vi "RFmx_MeasTest_Fetch.vi"(6 "RFmx_Data":refnum<queue>, 7 "Meas_Type":string[](array[string]), 8 "error in (no error)":errorcluster, 11 "Instrument Handle in":refnum<k21>) -> (0 "error out":errorcluster, 3 "Instrument Handle out":refnum<k21>)   [LabVIEW 2014]
uses:
  02_Controls/Message_Data_Ctl.ctl
  <vilib>/RFmx/RFInstr/mx/RFmxInstr.llb/RFmxInstr Build Signal String.vi
  <vilib>/RFmx/SpecAn/mx/RFmxSpecAn.llb/RFmxSpecAn Spectrum Fetch Measurement.vi
  <vilib>/RFmx/SpecAn/mx/RFmxSpecAn.llb/RFmxSpecAn Spectrum Fetch Spectrum.vi
  <vilib>/RFmx/SpecAn/mx/RFmxSpecAn.llb/RFmxSpecAn ACP Fetch Total Carrier Power.vi
  <vilib>/RFmx/SpecAn/mx/RFmxSpecAn.llb/RFmxSpecAn ACP Fetch Offset Measurement (Array).vi
  <vilib>/RFmx/SpecAn/mx/RFmxSpecAn.llb/RFmxSpecAn ACP Fetch Spectrum.vi
  <vilib>/RFmx/SpecAn/mx/RFmxSpecAn.llb/RFmxSpecAn CHP Fetch Total Carrier Power.vi
  <vilib>/RFmx/SpecAn/mx/RFmxSpecAn.llb/RFmxSpecAn CHP Fetch Spectrum.vi
  <vilib>/RFmx/SpecAn/mx/RFmxSpecAn.llb/RFmxSpecAn OBW Fetch Measurement.vi
  <vilib>/RFmx/SpecAn/mx/RFmxSpecAn.llb/RFmxSpecAn OBW Fetch Spectrum Trace.vi
  <vilib>/RFmx/SpecAn/mx/RFmxSpecAn.llb/RFmxSpecAn TXP Fetch Measurement.vi
  <vilib>/RFmx/SpecAn/mx/RFmxSpecAn.llb/RFmxSpecAn TXP Fetch Power Trace.vi
  <vilib>/RFmx/SpecAn/mx/RFmxSpecAn.llb/RFmxSpecAn CCDF Fetch Power.vi
  <vilib>/RFmx/SpecAn/mx/RFmxSpecAn.llb/RFmxSpecAn CCDF Fetch Probabilities Trace.vi
  <vilib>/RFmx/SpecAn/mx/RFmxSpecAn.llb/RFmxSpecAn CCDF Fetch Gaussian Probabilities Trace.vi
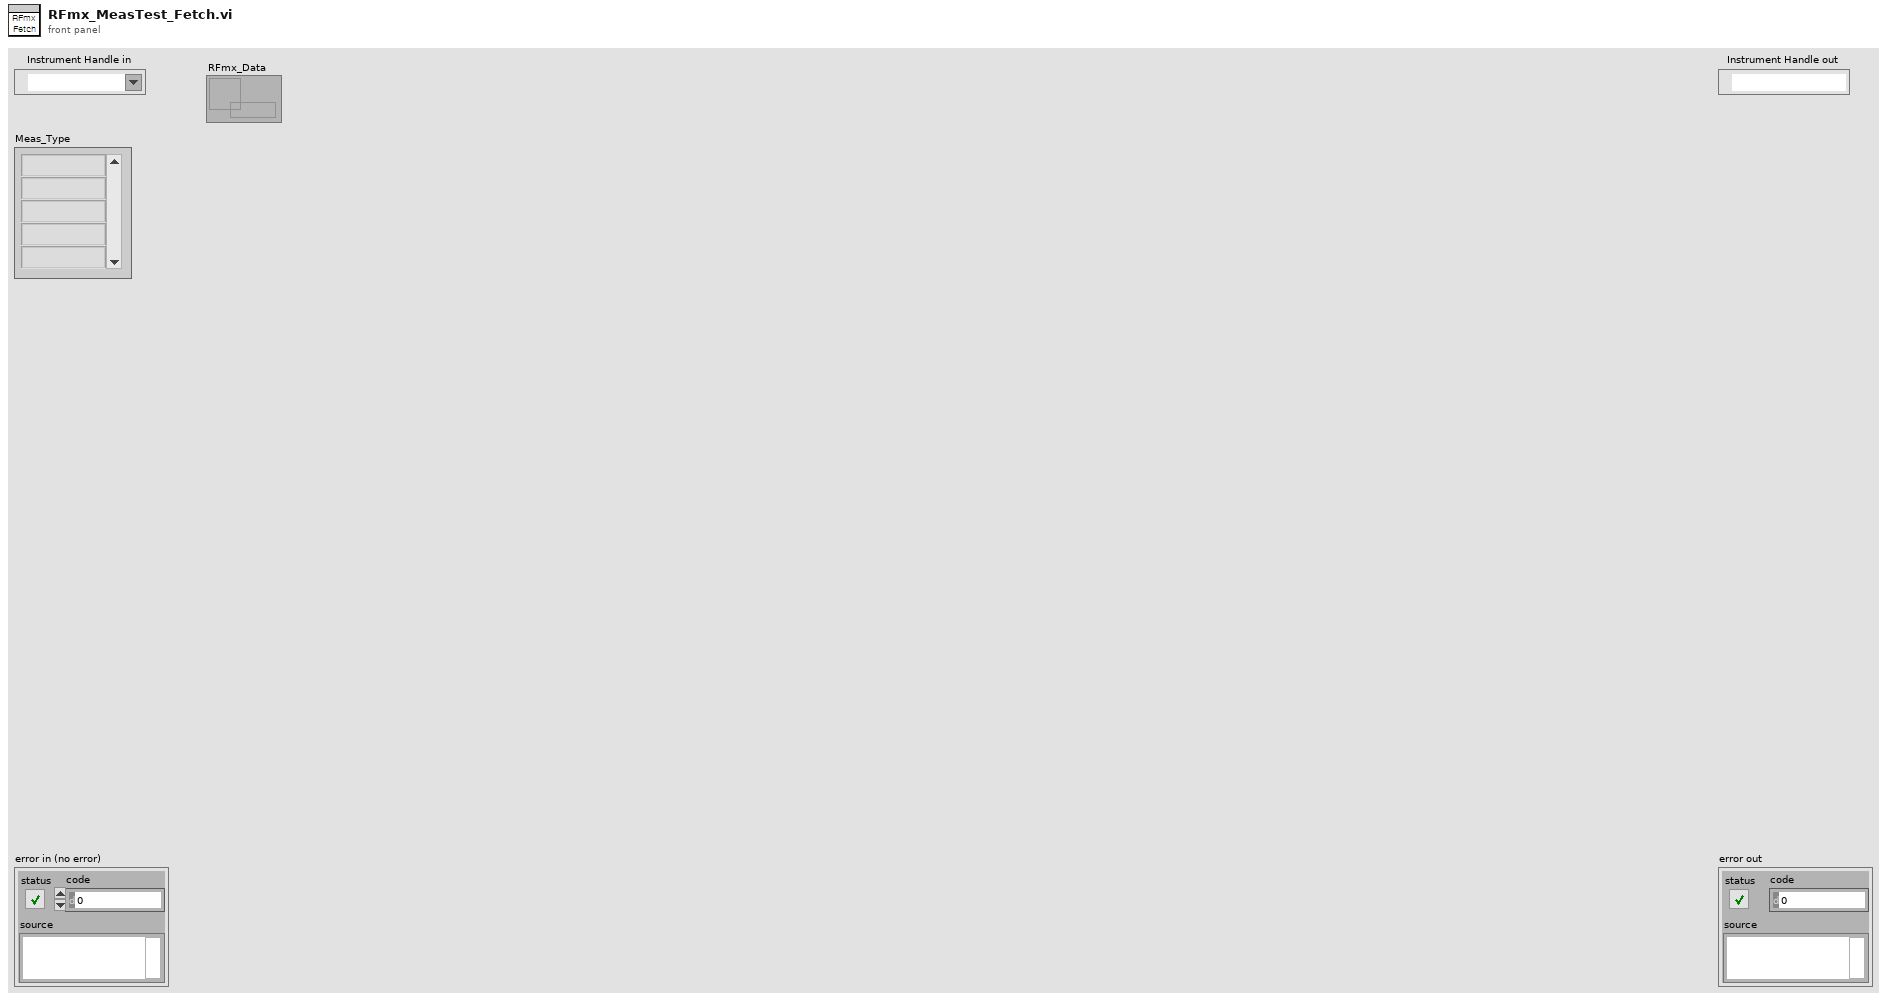
[diagram p1: front panel]
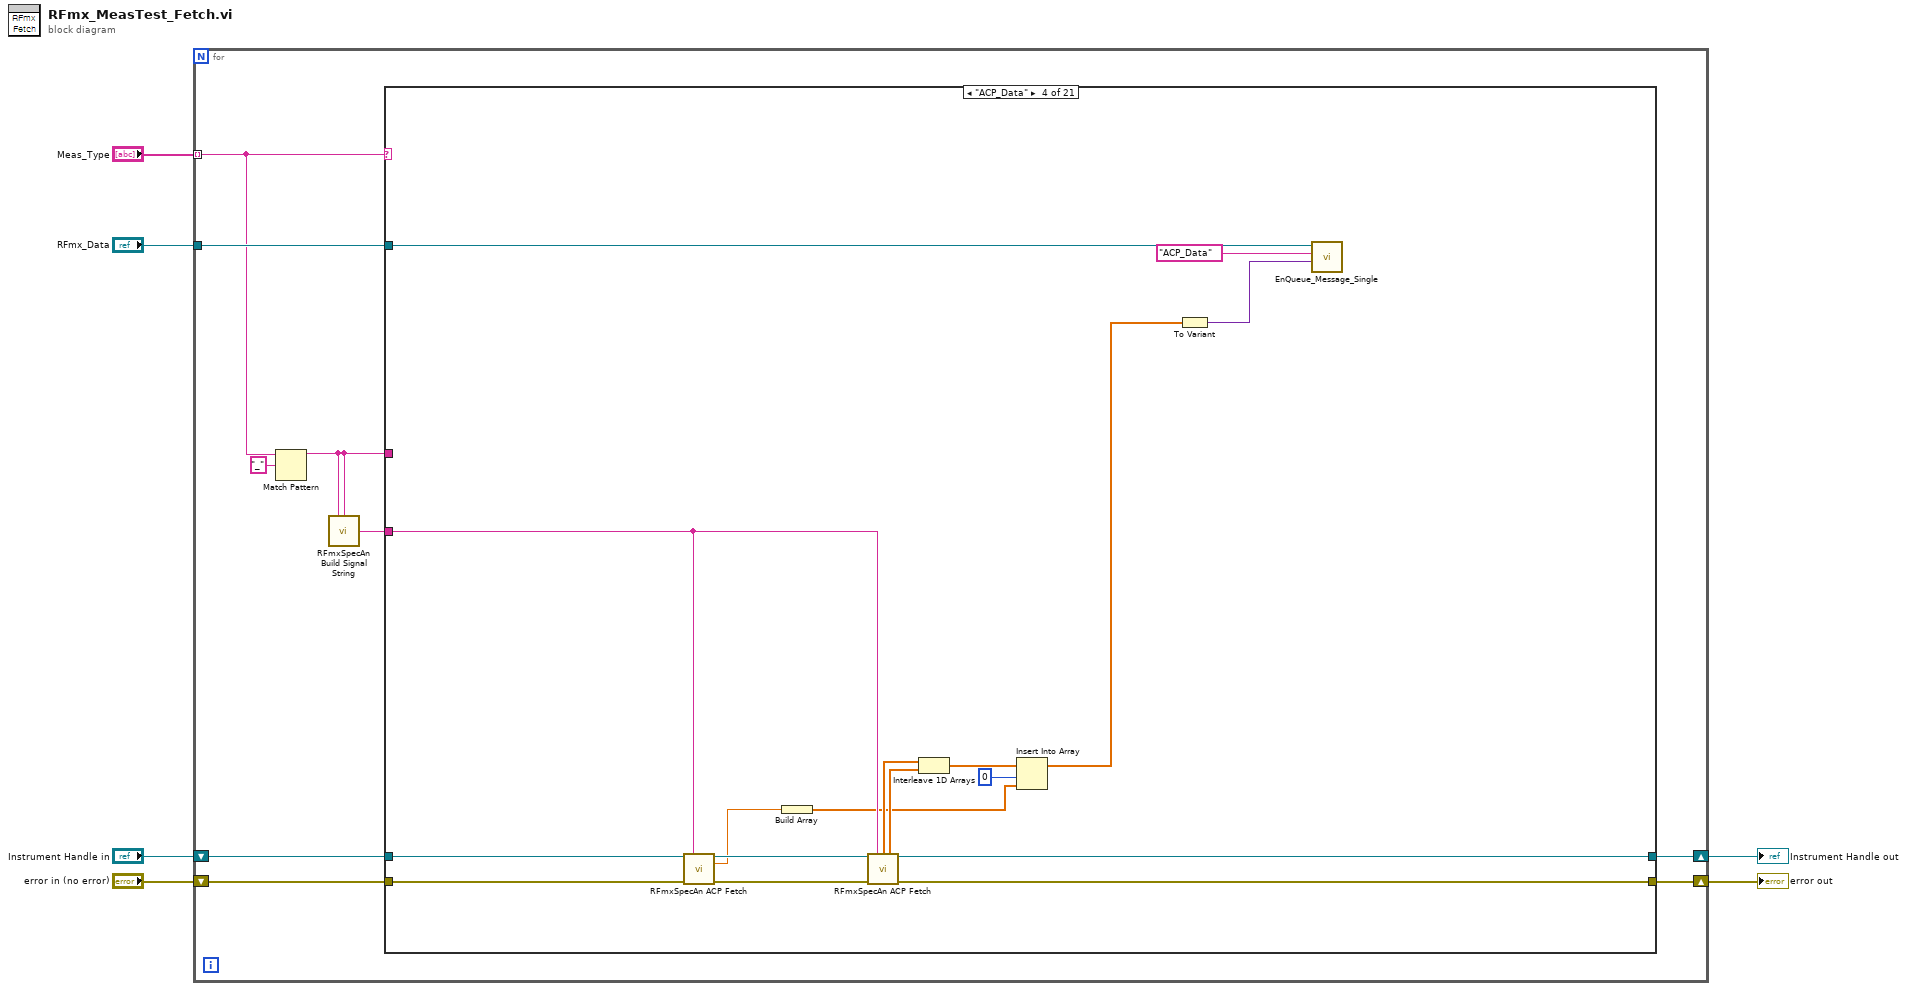
[diagram p0: block diagram]
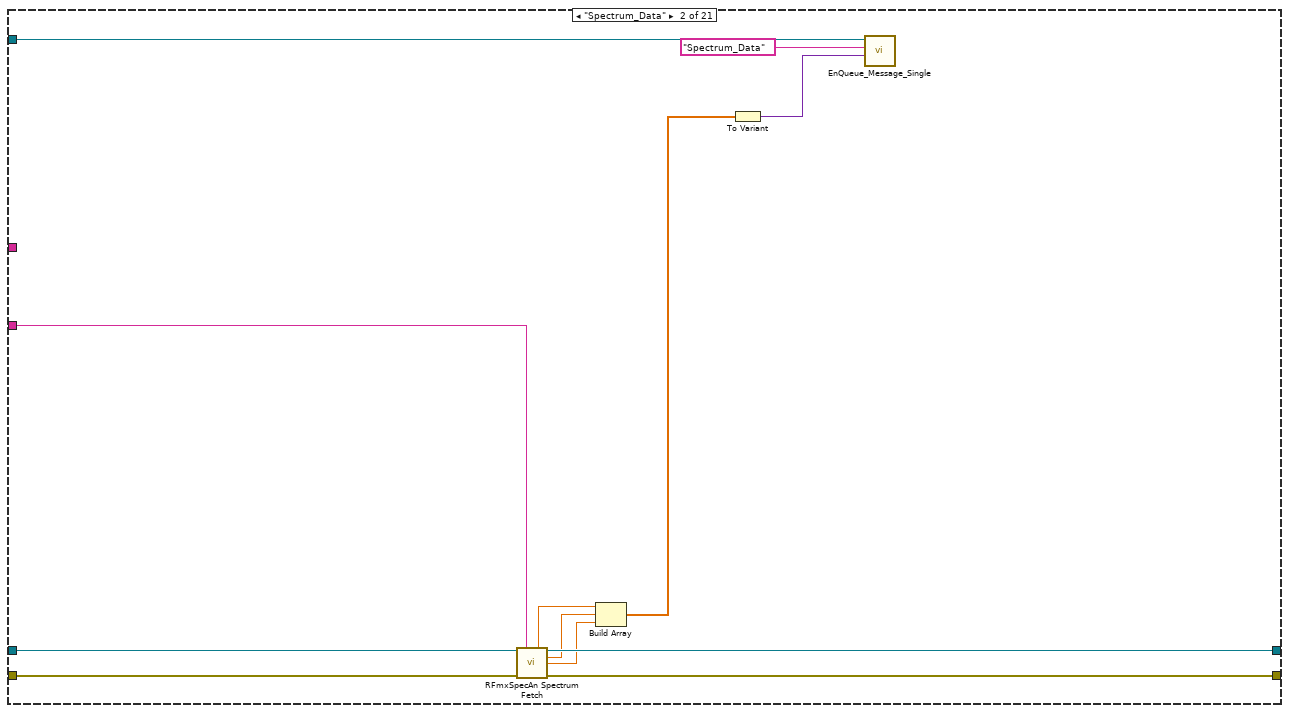
[diagram p3: hidden frame]
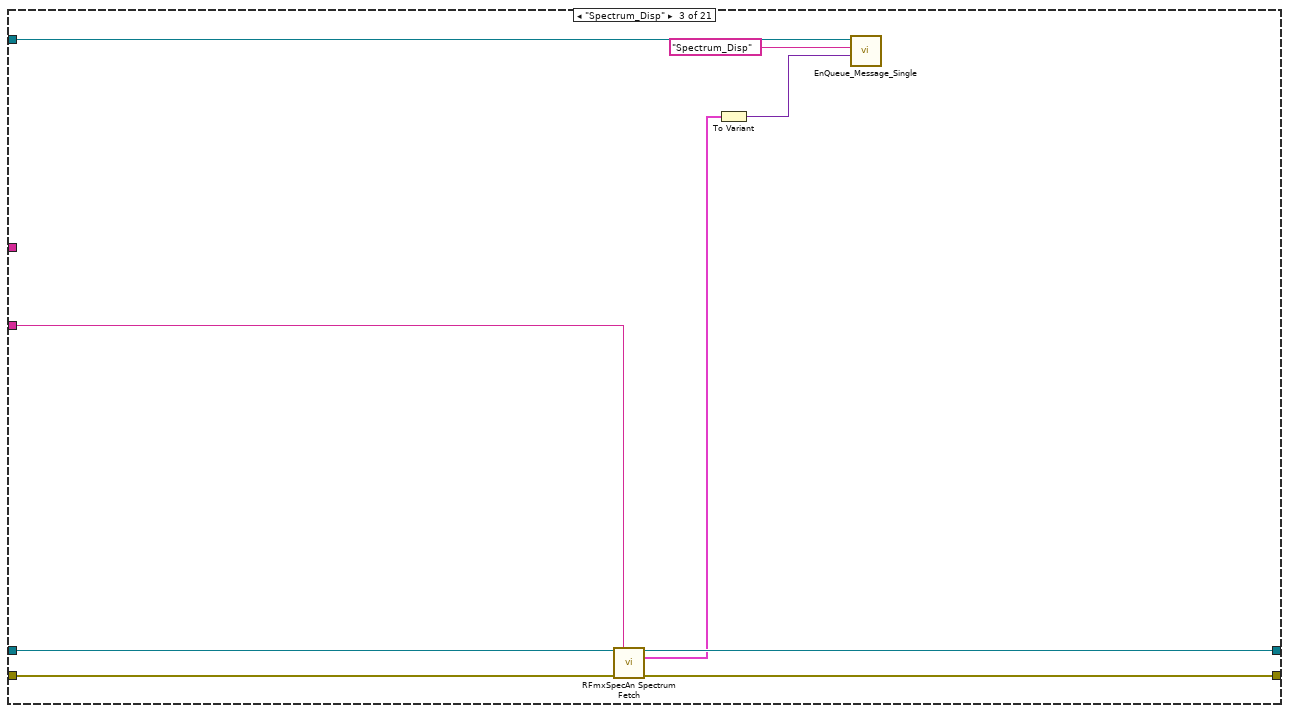
[diagram p4: hidden frame]
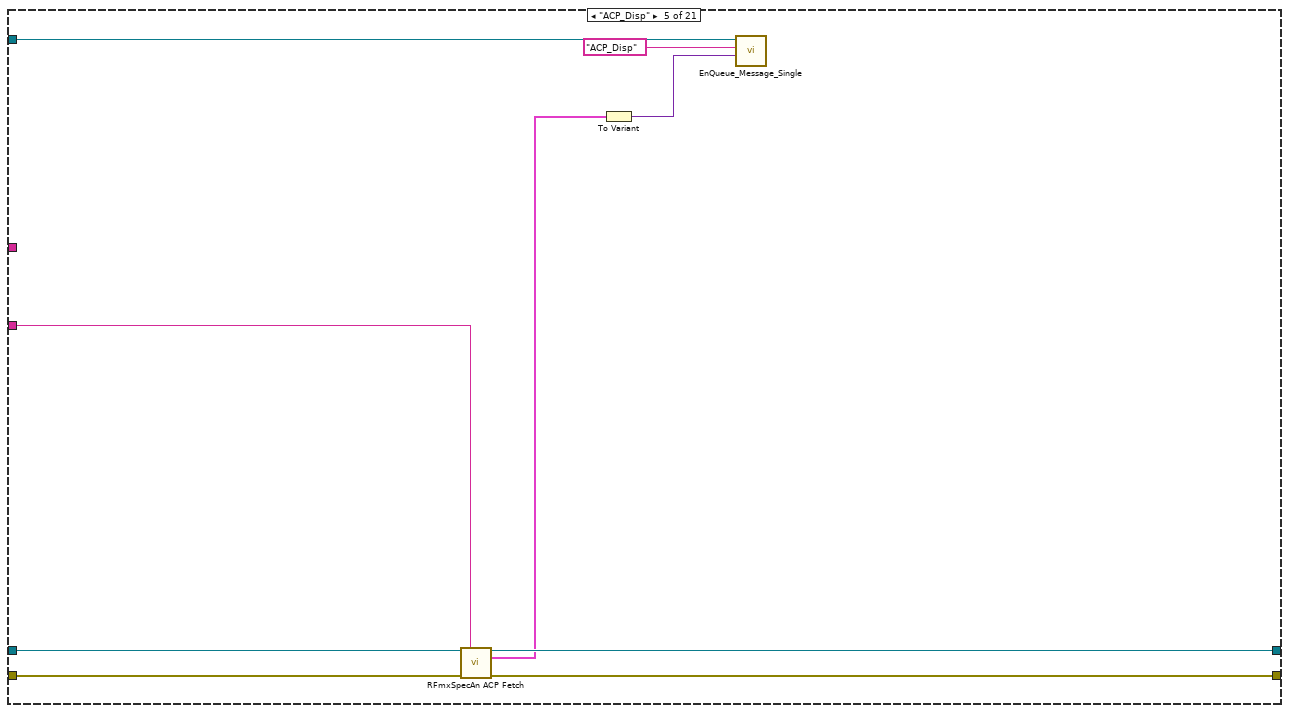
[diagram p5: hidden frame]
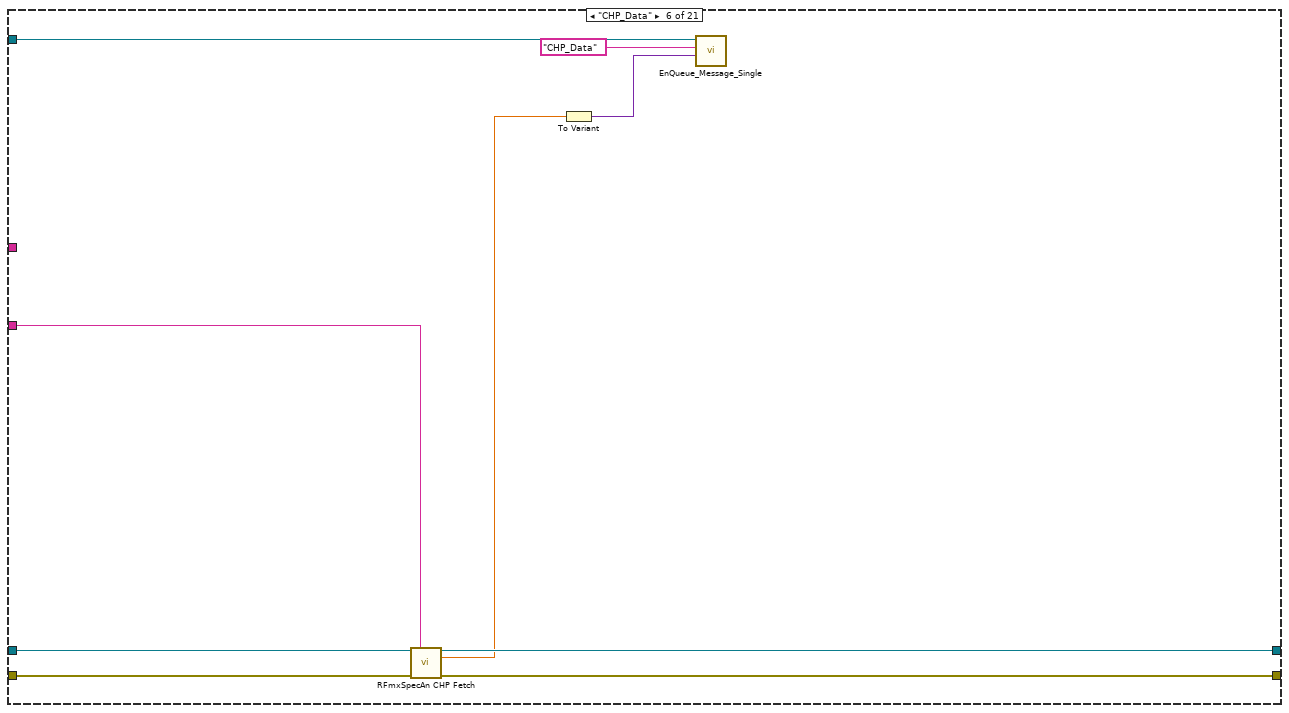
[diagram p6: hidden frame]
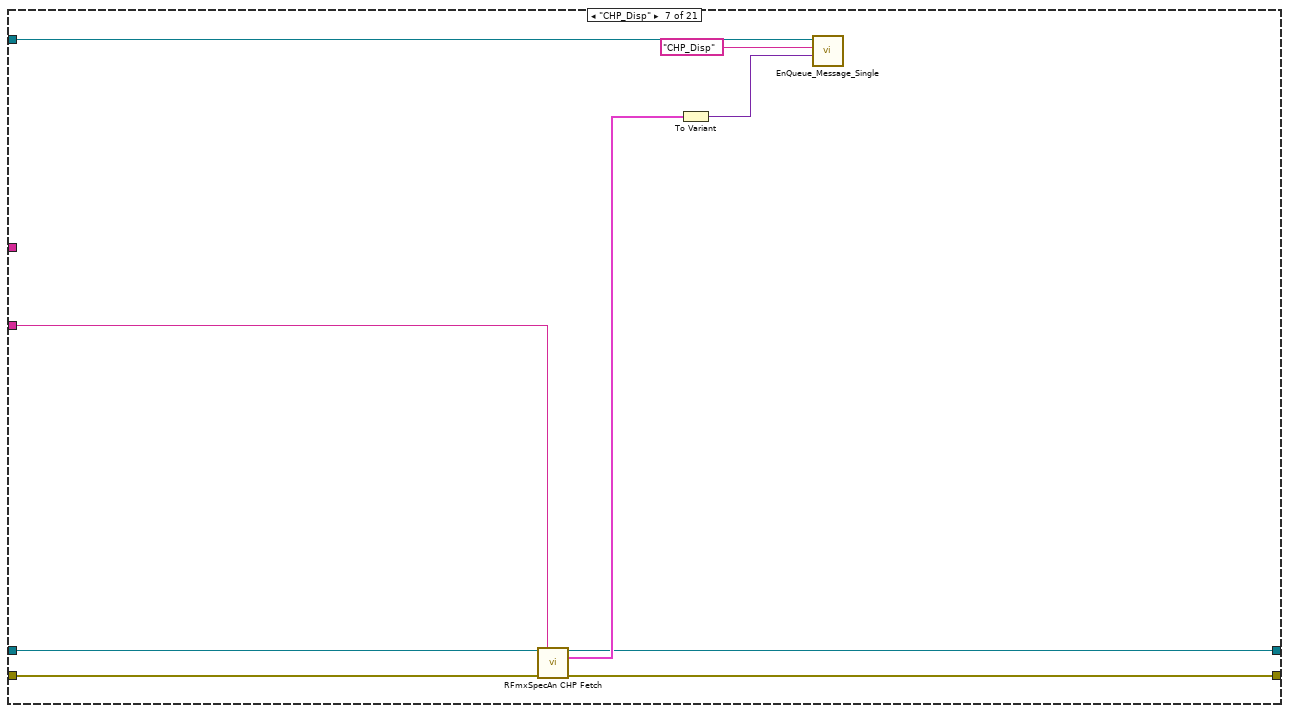
[diagram p7: hidden frame]
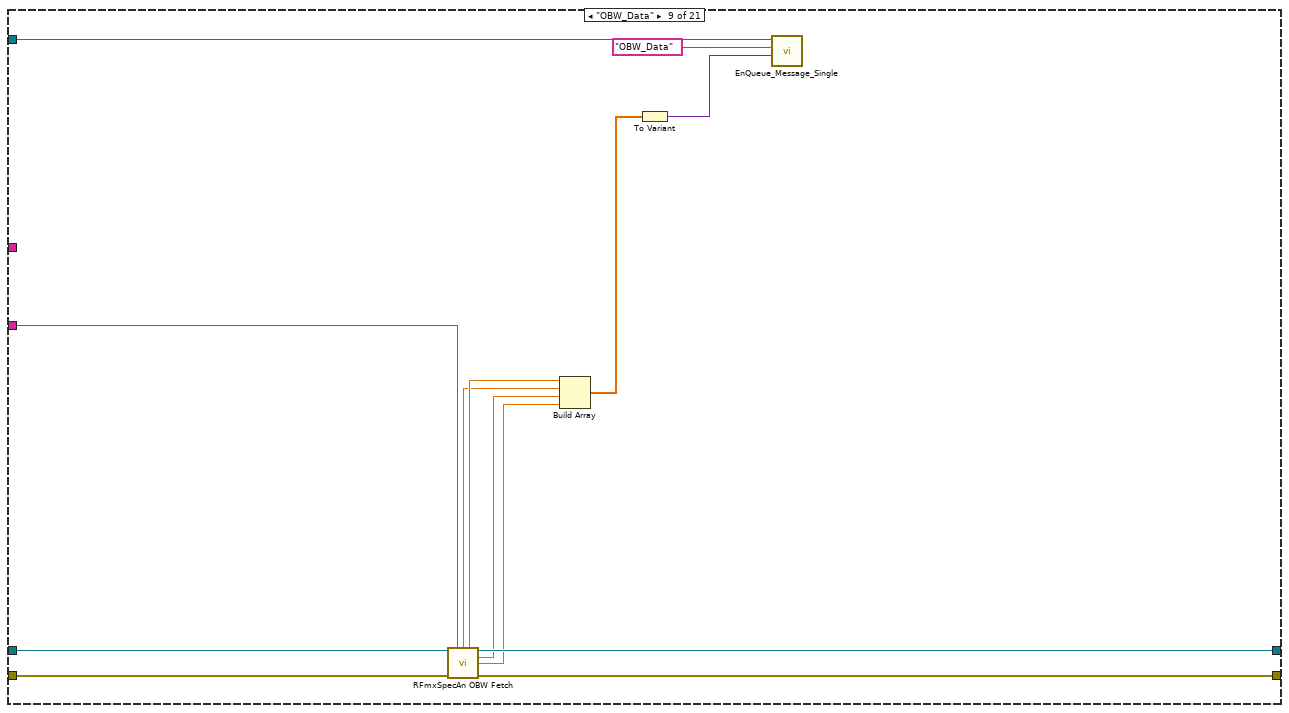
[diagram p9: hidden frame]
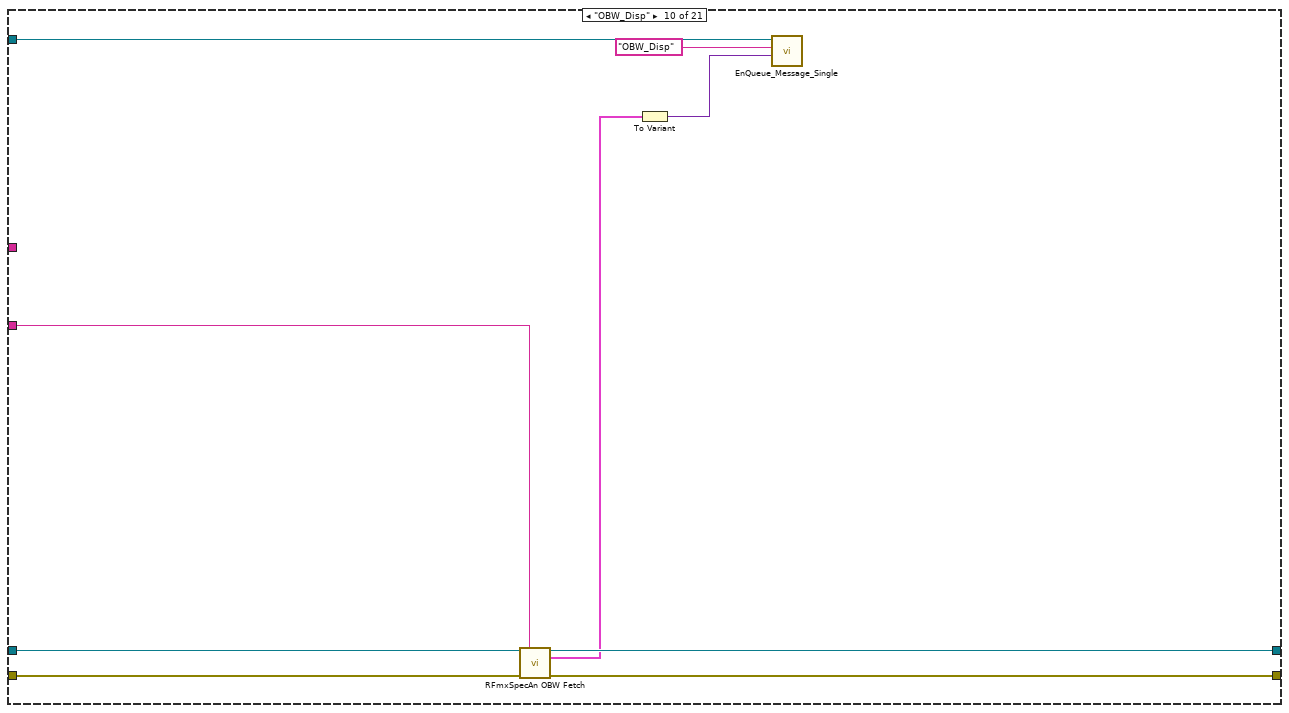
[diagram p10: hidden frame]
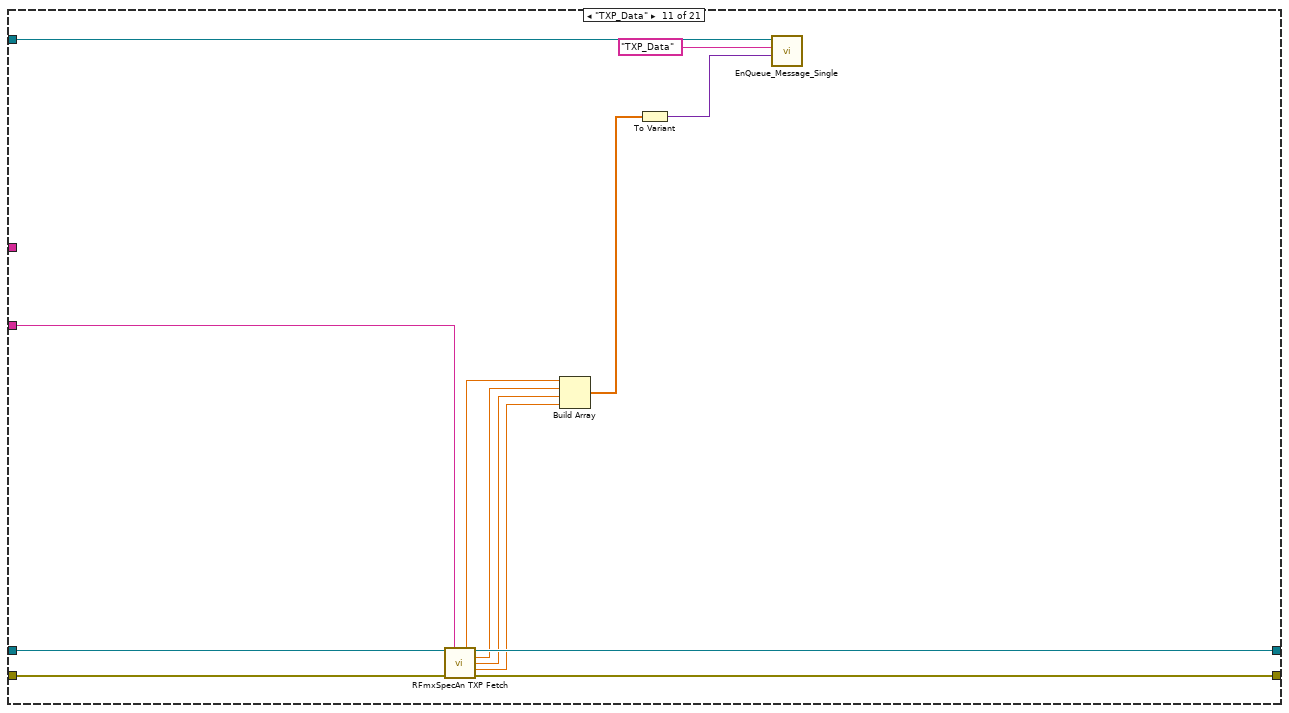
[diagram p11: hidden frame]
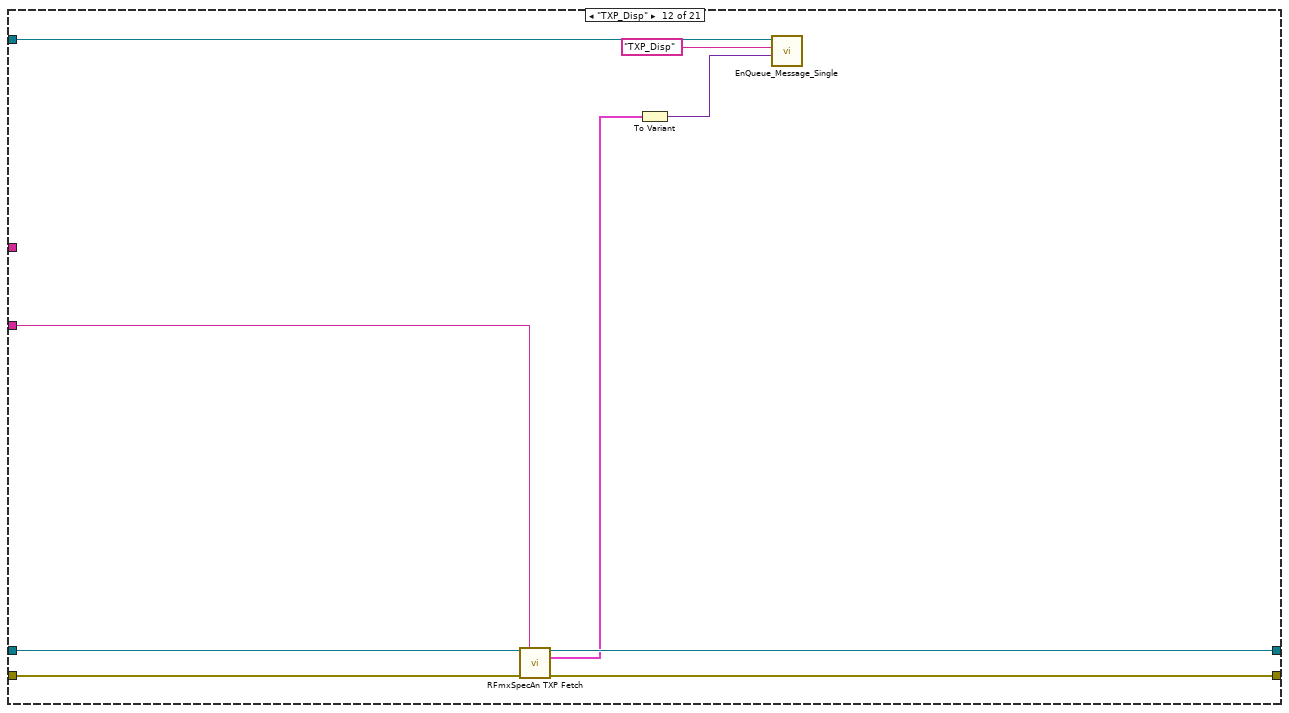
[diagram p12: hidden frame]
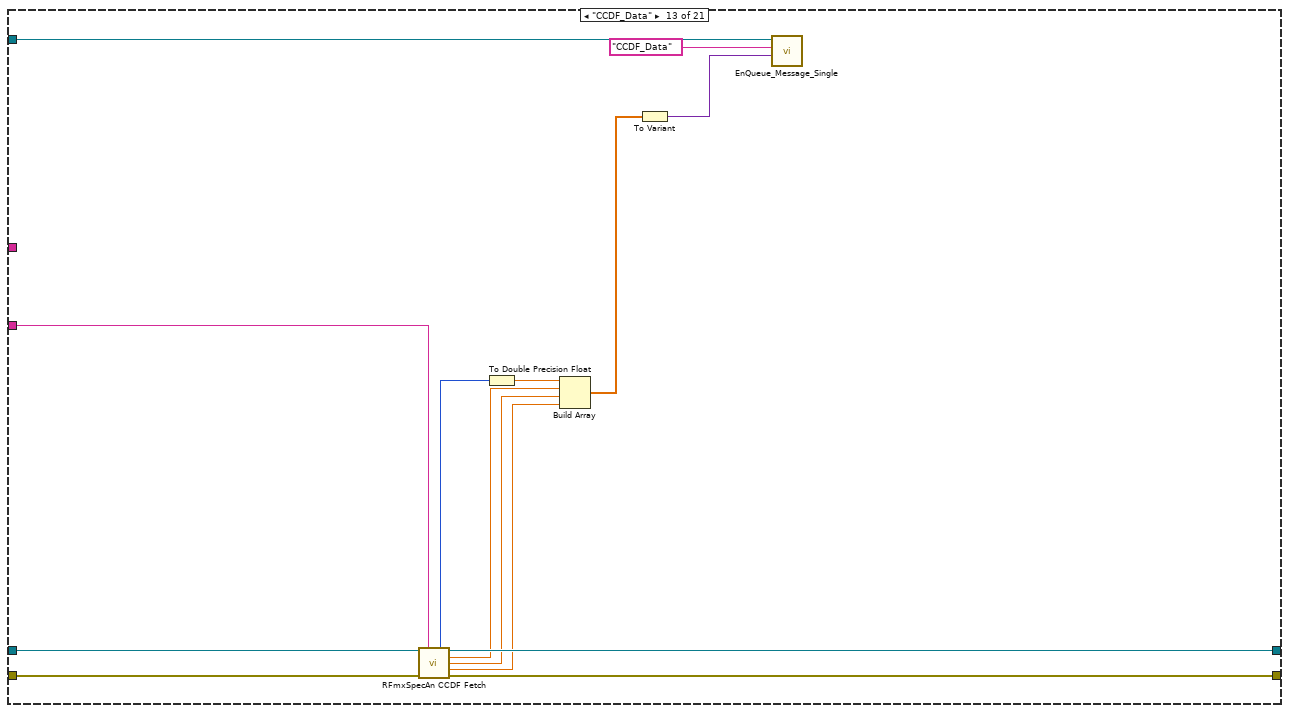
[diagram p13: hidden frame]
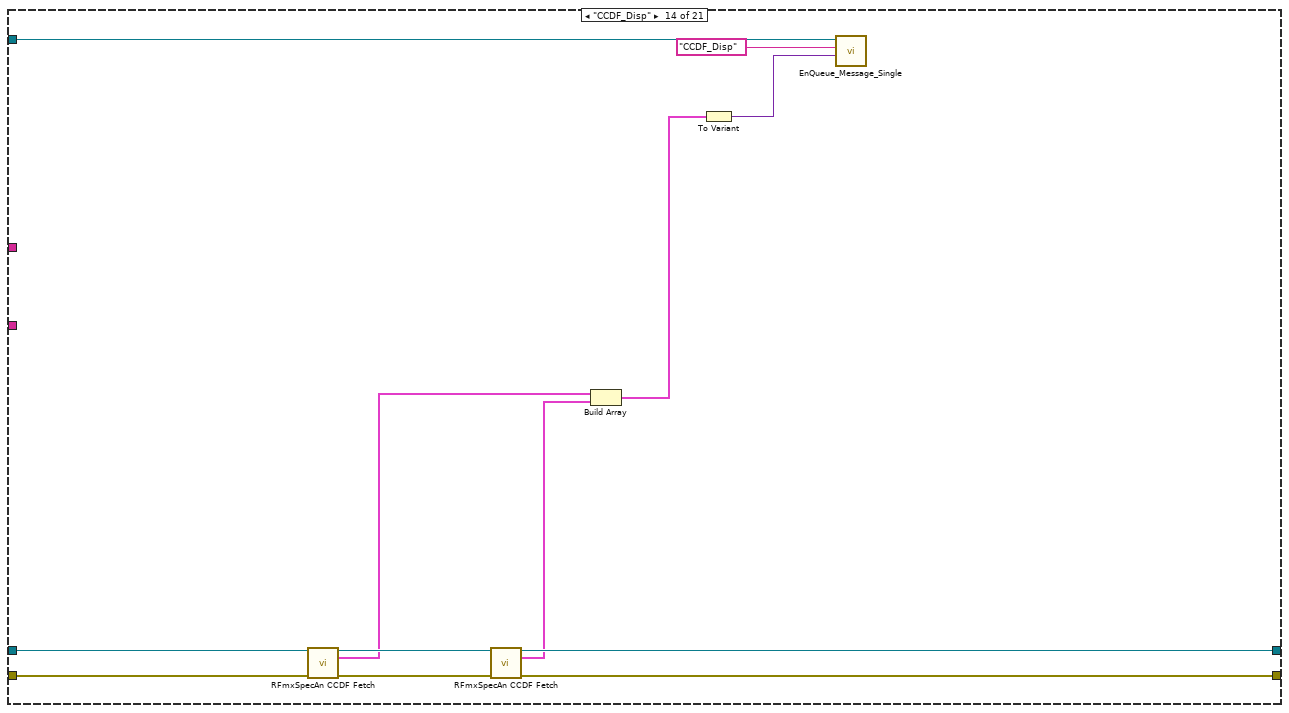
[diagram p14: hidden frame]
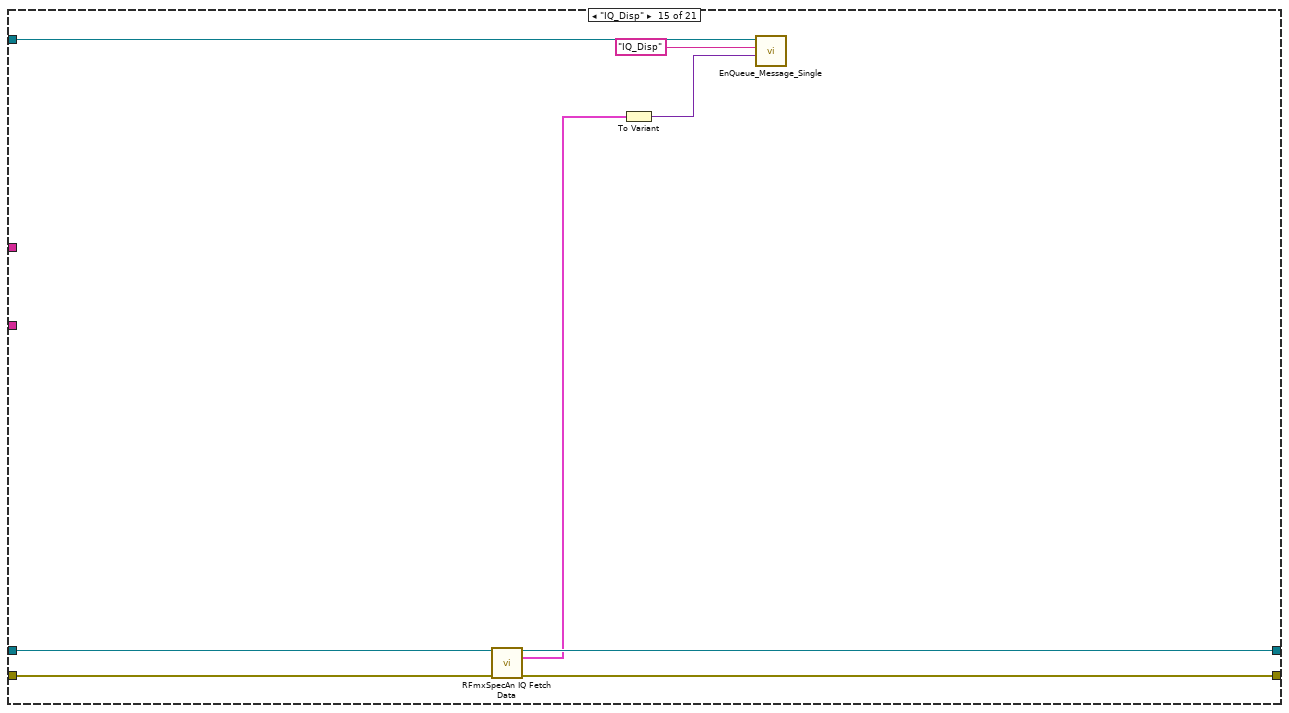
[diagram p15: hidden frame]
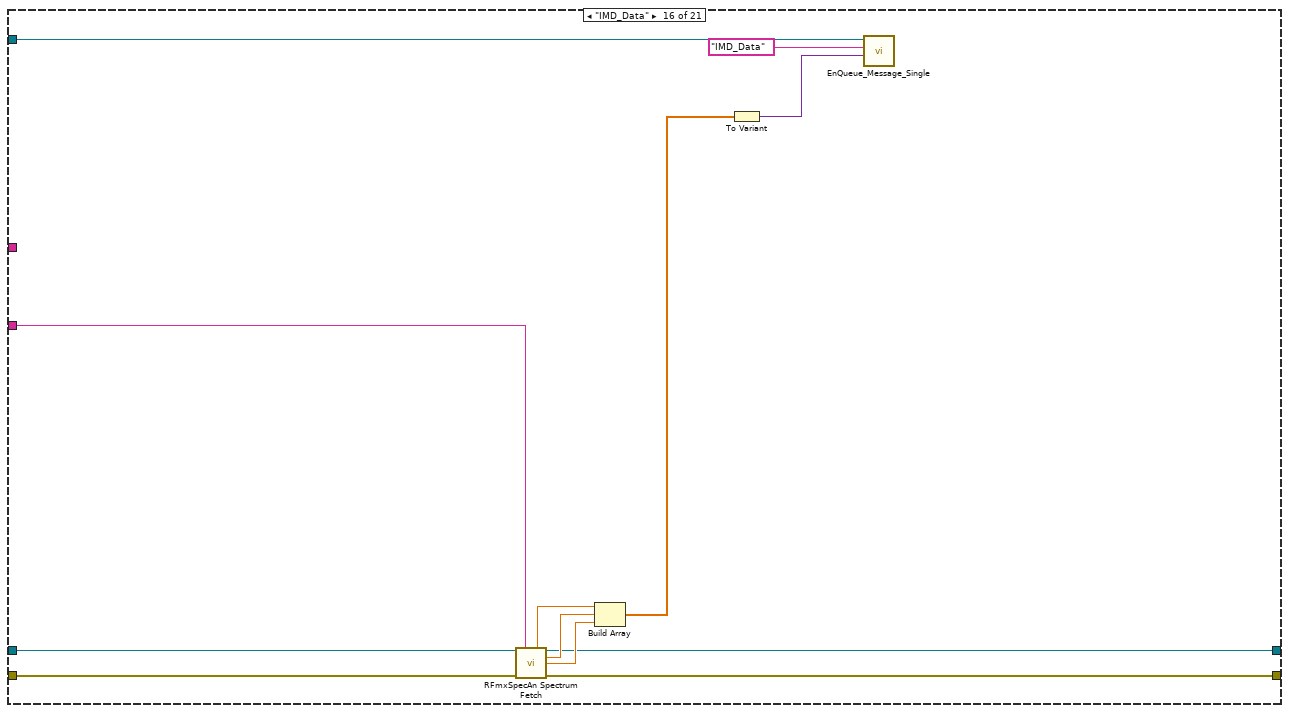
[diagram p16: hidden frame]
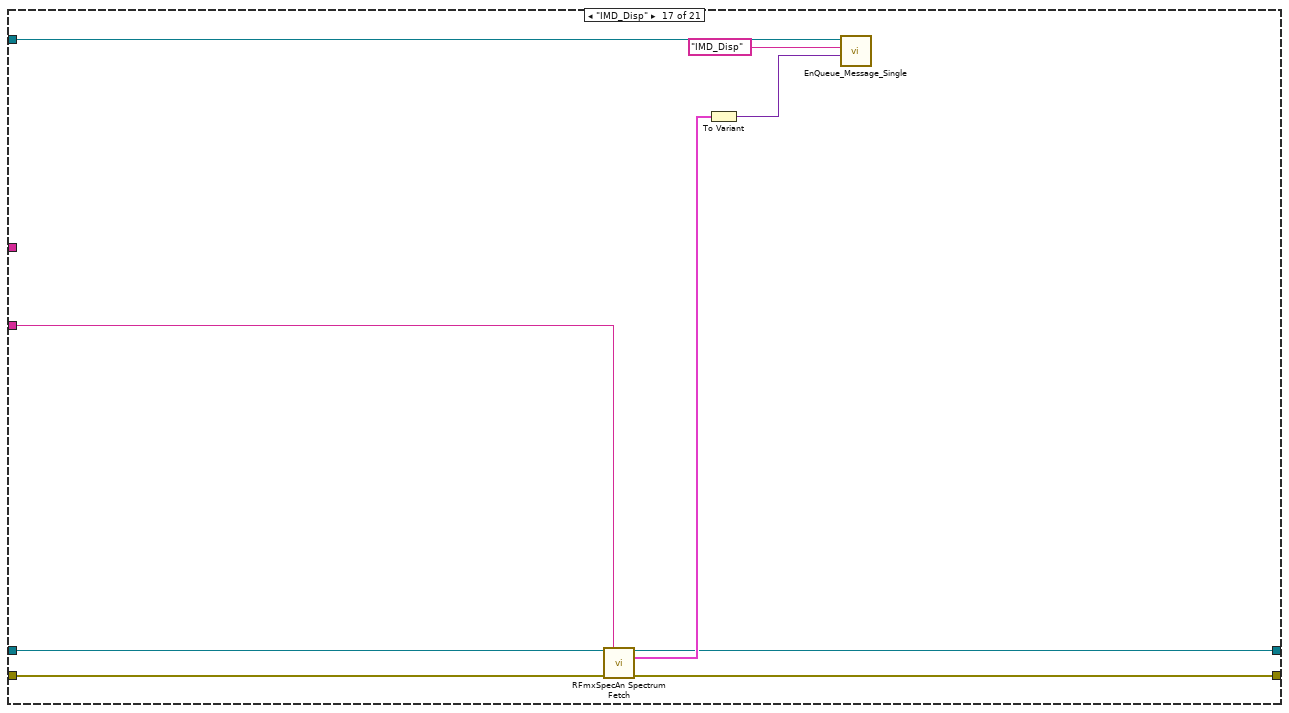
[diagram p17: hidden frame]
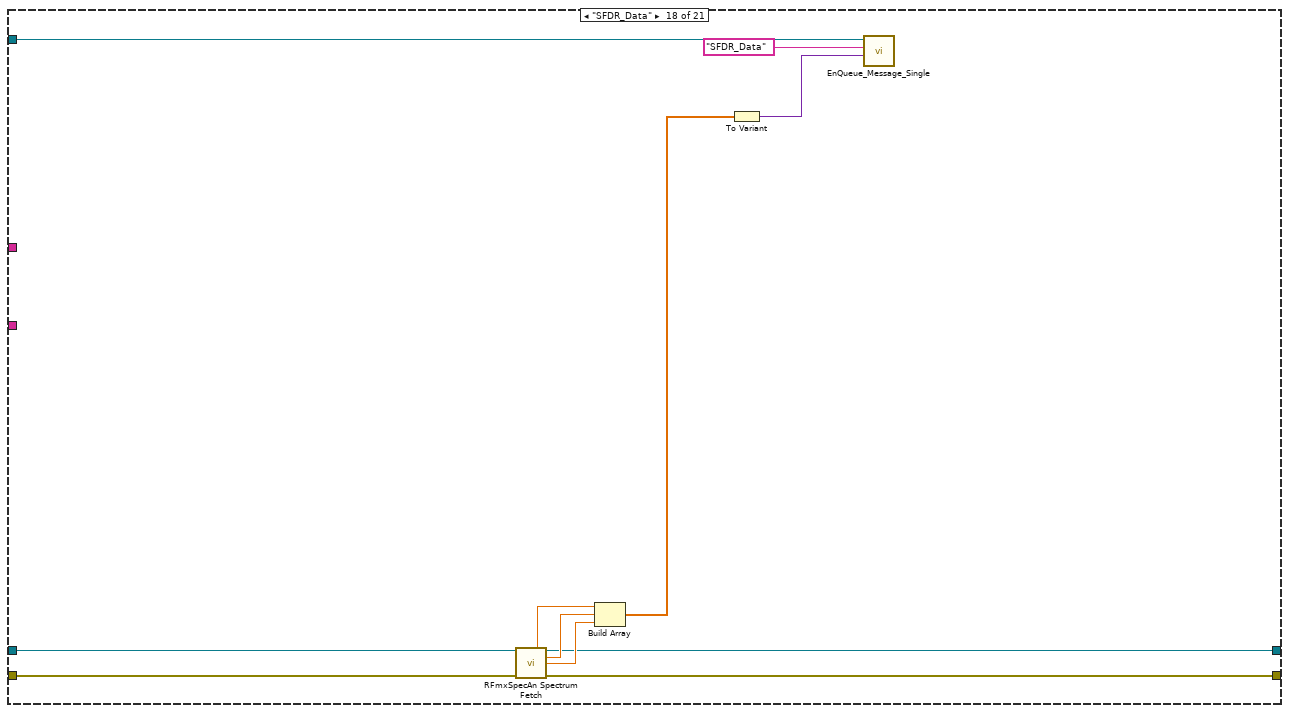
[diagram p18: hidden frame]
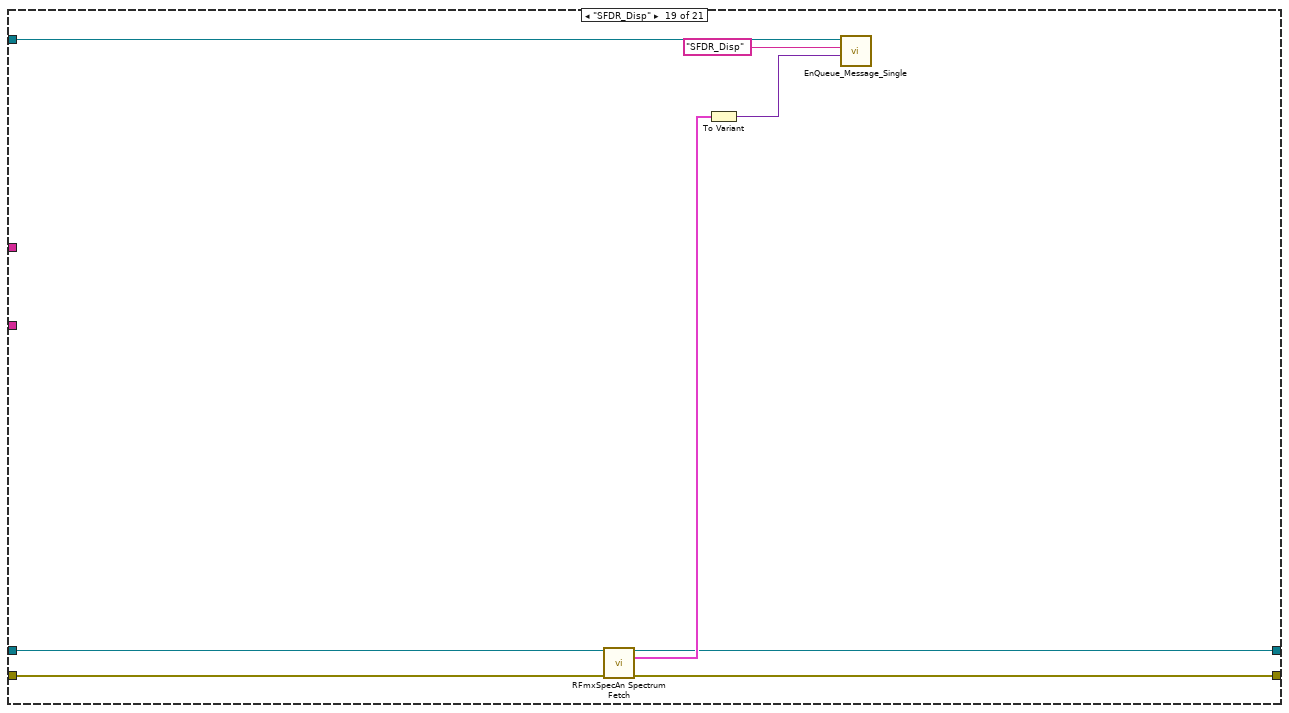
[diagram p19: hidden frame]
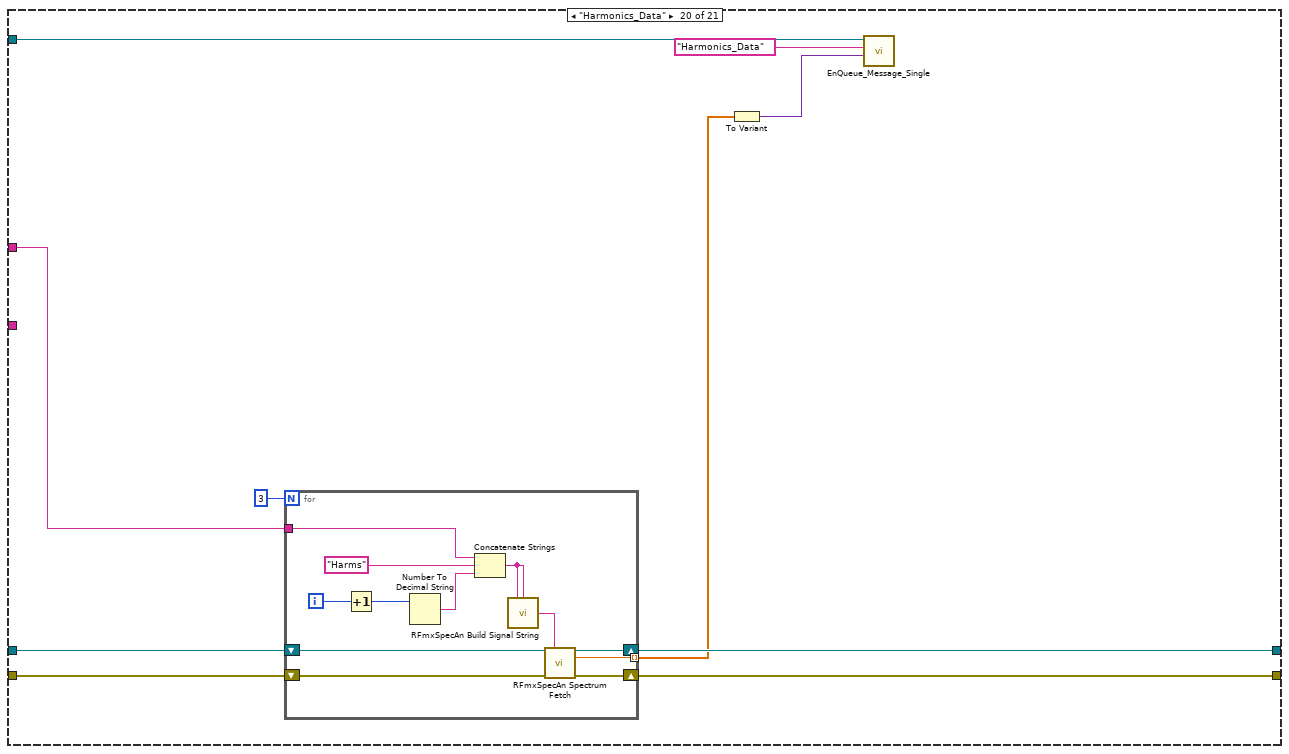
[diagram p20: hidden frame]
diagram:
  n1 = for {
    tunnel: "RFmx_Data" -> [w11]
    shift-right: [w12] -> w3
    shift-left: "Instrument Handle in" -> [w15]
    shift-right: [w13] -> w4
    shift-left: "error in (no error)" -> [w14]
    tunnel: "Meas_Type" -> [w8] mode=indexing
    n2 = Match Pattern(string=w8, regular expression="_") -> (before substring=w7:string)  [unwired: 1 in, 3 out]
    n3 = call <vilib>:"RFmxSpecAn Build Signal String.vi"("Signal Name"=w7, "Result Name"=w7) -> ("Selector String"=w10:string)  [unwired: 13 in]
    n4 = case shown="\"ACP_Data\"" w8 {
      tunnel: w15 -> [w17 w29 w38 w54 w58 w68 w79 w84 w97 w106 w115 w128 w138 w149 w162 w168 w180 w188 w199 w207 w230]
      tunnel: w14 -> [w16 w28 w37 w53 w57 w67 w78 w83 w96 w105 w114 w127 w137 w148 w161 w167 w179 w187 w198 w206 w229]
      tunnel: [w17 w27 w36 w50 w64 w70 w76 w84 w95 w104 w112 w126 w135 w151 w160 w166 w177 w186 w196 w205 w228] -> w12
      tunnel: [w16 w26 w35 w49 w63 w69 w77 w83 w94 w103 w113 w125 w136 w150 w159 w165 w176 w185 w195 w204 w227] -> w13
      tunnel: w11 -> [_ w23 w31 w55 w61 w73 w75 _ w91 w100 w117 w122 w140 w152 w156 w164 w178 w184 w197 w210 w232]
      tunnel: w10 -> [_ w18 w30 w41 w56 w65 w74 _ w85 w98 w107 w120 w129 _ _ w163 w175 _ _ _ _]
      tunnel: w7 -> [_ _ _ _ _ _ _ _ _ _ _ _ _ _ _ _ _ _ _ w208 w226]
      frame "Nothing", Default {
      }
      frame "Spectrum_Data" {
        n5 = call-poly <vilib>:"RFmxSpecAn Spectrum Fetch.vi"("Instrument Handle In"=w29, "Selector String"=w18, "error in (no error)"=w28) -> ("Frequency Resolution (Hz)"=w22:dbl, "Instrument Handle Out"=w27:refnum<k21>, "Peak Amplitude"=w21:dbl, "Peak Frequency (Hz)"=w20:dbl, "error out"=w26:errorcluster)  [unwired: 8 in]
        n6 = Build Array(w22, w21, w20) -> (w19:dbl[])
        n7 = To Variant(anything=w19) -> (Variant=w25:variant)
        n8 = call "EnQueue_Message_Single.vi"("Message Data"=w25, "Message"="Spectrum_Data", "Message_Queue"=w23) -> ()  [unwired: 7 in, 2 out]
      }
      frame "Spectrum_Disp" {
        n9 = call-poly <vilib>:"RFmxSpecAn Spectrum Fetch.vi"("Instrument Handle In"=w38, "Selector String"=w30, "error in (no error)"=w37) -> ("Instrument Handle Out"=w36:refnum<k21>, "Spectrum"=w32:cluster{"x0":dbl, "dx":dbl, "y":sgl[]}, "error out"=w35:errorcluster)  [unwired: 10 in]
        n10 = To Variant(anything=w32) -> (Variant=w34:variant)
        n11 = call "EnQueue_Message_Single.vi"("Message Data"=w34, "Message"="Spectrum_Disp", "Message_Queue"=w31) -> ()  [unwired: 7 in, 2 out]
      }
      frame "ACP_Data" {
        n12 = call-poly <vilib>:"RFmxSpecAn ACP Fetch.vi"("Instrument Handle In"=w54, "Selector String"=w41, "error in (no error)"=w53) -> ("Instrument Handle Out"=w52:refnum<k21>, "Total Carrier Power (dBm or dBm/Hz)"=w44:dbl, "error out"=w51:errorcluster)  [unwired: 10 in]
        n13 = Build Array(w44) -> (w39:dbl[])
        n14 = call-poly <vilib>:"RFmxSpecAn ACP Fetch.vi"("Instrument Handle In"=w52, "Selector String"=w41, "error in (no error)"=w51) -> ("Lower Absolute Power (dBm or dBm/Hz)"=w46:dbl[], "Upper Absolute Power (dBm or dBm/Hz)"=w45:dbl[], "Instrument Handle Out"=w50:refnum<k21>, "error out"=w49:errorcluster)  [unwired: 7 in, 2 out]
        n15 = Interleave 1D Arrays(w46, w45) -> (w40:dbl[])
        n16 = Insert Into Array(array=w40, index=0, new element=w39) -> (w42:dbl[])
        n17 = To Variant(anything=w42) -> (Variant=w48:variant)
        n18 = call "EnQueue_Message_Single.vi"("Message Data"=w48, "Message"="ACP_Data", "Message_Queue"=w55) -> ()  [unwired: 7 in, 2 out]
      }
      frame "ACP_Disp" {
        n19 = call-poly <vilib>:"RFmxSpecAn ACP Fetch.vi"("Instrument Handle In"=w58, "Selector String"=w56, "error in (no error)"=w57) -> ("Instrument Handle Out"=w64:refnum<k21>, "Spectrum (dBm or dBm/Hz)"=w62:cluster{"x0":dbl, "dx":dbl, "y":sgl[]}, "error out"=w63:errorcluster)  [unwired: 10 in]
        n20 = To Variant(anything=w62) -> (Variant=w60:variant)
        n21 = call "EnQueue_Message_Single.vi"("Message Data"=w60, "Message"="ACP_Disp", "Message_Queue"=w61) -> ()  [unwired: 7 in, 2 out]
      }
      frame "CHP_Data" {
        n22 = call-poly <vilib>:"RFmxSpecAn CHP Fetch.vi"("Instrument Handle In"=w68, "Selector String"=w65, "error in (no error)"=w67) -> ("Instrument Handle Out"=w70:refnum<k21>, "Total Carrier Power (dBm)"=w66:dbl, "error out"=w69:errorcluster)  [unwired: 10 in]
        n23 = To Variant(anything=w66) -> (Variant=w72:variant)
        n24 = call "EnQueue_Message_Single.vi"("Message Data"=w72, "Message"="CHP_Data", "Message_Queue"=w73) -> ()  [unwired: 7 in, 2 out]
      }
      frame "CHP_Disp" {
        n25 = call-poly <vilib>:"RFmxSpecAn CHP Fetch.vi"("Instrument Handle In"=w79, "Selector String"=w74, "error in (no error)"=w78) -> ("Instrument Handle Out"=w76:refnum<k21>, "Spectrum (dBm)"=w82:cluster{"x0":dbl, "dx":dbl, "y":sgl[]}, "error out"=w77:errorcluster)  [unwired: 10 in]
        n26 = To Variant(anything=w82) -> (Variant=w81:variant)
        n27 = call "EnQueue_Message_Single.vi"("Message Data"=w81, "Message"="CHP_Disp", "Message_Queue"=w75) -> ()  [unwired: 7 in, 2 out]
      }
      frame "FCnt" {
      }
      frame "OBW_Data" {
        n28 = call-poly <vilib>:"RFmxSpecAn OBW Fetch.vi"("Instrument Handle In"=w97, "Selector String"=w85, "error in (no error)"=w96) -> ("Stop Frequency (Hz)"=w89:dbl, "Start Frequency (Hz)"=w90:dbl, "Instrument Handle Out"=w95:refnum<k21>, "Occupied Bandwidth (Hz)"=w88:dbl, "Average Power (dBm or dBm/Hz)"=w87:dbl, "error out"=w94:errorcluster)  [unwired: 6 in, 1 out]
        n29 = Build Array(w90, w89, w88, w87) -> (w86:dbl[])
        n30 = To Variant(anything=w86) -> (Variant=w93:variant)
        n31 = call "EnQueue_Message_Single.vi"("Message Data"=w93, "Message"="OBW_Data", "Message_Queue"=w91) -> ()  [unwired: 7 in, 2 out]
      }
      frame "OBW_Disp" {
        n32 = call-poly <vilib>:"RFmxSpecAn OBW Fetch.vi"("Instrument Handle In"=w106, "Selector String"=w98, "error in (no error)"=w105) -> ("Instrument Handle Out"=w104:refnum<k21>, "Spectrum (dBm)"=w99:cluster{"x0":dbl, "dx":dbl, "y":sgl[]}, "error out"=w103:errorcluster)  [unwired: 10 in]
        n33 = To Variant(anything=w99) -> (Variant=w102:variant)
        n34 = call "EnQueue_Message_Single.vi"("Message Data"=w102, "Message"="OBW_Disp", "Message_Queue"=w100) -> ()  [unwired: 7 in, 2 out]
      }
      frame "TXP_Data" {
        n35 = call-poly <vilib>:"RFmxSpecAn TXP Fetch.vi"("Instrument Handle In"=w115, "Selector String"=w107, "error in (no error)"=w114) -> ("Minimum Power (dBm)"=w111:dbl, "Instrument Handle Out"=w112:refnum<k21>, "Average Mean Power (dBm)"=w110:dbl, "Peak to Average Ratio (dB)"=w109:dbl, "Maximum Power (dBm)"=w108:dbl, "error out"=w113:errorcluster)  [unwired: 7 in]
        n36 = Build Array(w111, w110, w109, w108) -> (w116:dbl[])
        n37 = To Variant(anything=w116) -> (Variant=w119:variant)
        n38 = call "EnQueue_Message_Single.vi"("Message Data"=w119, "Message"="TXP_Data", "Message_Queue"=w117) -> ()  [unwired: 7 in, 2 out]
      }
      frame "TXP_Disp" {
        n39 = call-poly <vilib>:"RFmxSpecAn TXP Fetch.vi"("Instrument Handle In"=w128, "Selector String"=w120, "error in (no error)"=w127) -> ("Instrument Handle Out"=w126:refnum<k21>, "Power (dBm)"=w121:cluster{"x0":dbl, "dx":dbl, "y":sgl[]}, "error out"=w125:errorcluster)  [unwired: 10 in]
        n40 = To Variant(anything=w121) -> (Variant=w124:variant)
        n41 = call "EnQueue_Message_Single.vi"("Message Data"=w124, "Message"="TXP_Disp", "Message_Queue"=w122) -> ()  [unwired: 7 in, 2 out]
      }
      frame "CCDF_Data" {
        n42 = call-poly <vilib>:"RFmxSpecAn CCDF Fetch.vi"("Instrument Handle In"=w138, "Selector String"=w129, "error in (no error)"=w137) -> ("Measured Samples Count"=w131:i32, "Instrument Handle Out"=w135:refnum<k21>, "Mean Power (dBm)"=w134:dbl, "Mean Power Percentile (%)"=w133:dbl, "Peak Power (dB)"=w132:dbl, "error out"=w136:errorcluster)  [unwired: 7 in]
        n43 = To Double Precision Float(number=w131) -> (double precision float=w130:dbl)
        n44 = Build Array(w130, w134, w133, w132) -> (w139:dbl[])
        n45 = To Variant(anything=w139) -> (Variant=w142:variant)
        n46 = call "EnQueue_Message_Single.vi"("Message Data"=w142, "Message"="CCDF_Data", "Message_Queue"=w140) -> ()  [unwired: 7 in, 2 out]
      }
      frame "CCDF_Disp" {
        n47 = call-poly <vilib>:"RFmxSpecAn CCDF Fetch.vi"("Instrument Handle In"=w149, "error in (no error)"=w148) -> ("Instrument Handle Out"=w146:refnum<k21>, "Probabilities (%)"=w145:cluster{"x0":dbl, "dx":dbl, "y":sgl[]}, "error out"=w147:errorcluster)  [unwired: 11 in]
        n48 = call-poly <vilib>:"RFmxSpecAn CCDF Fetch.vi"("Instrument Handle In"=w146, "error in (no error)"=w147) -> ("Instrument Handle Out"=w151:refnum<k21>, "Gaussian Probabilities (%)"=w144:cluster{"x0":dbl, "dx":dbl, "y":sgl[]}, "error out"=w150:errorcluster)  [unwired: 11 in]
        n49 = Build Array(w145, w144) -> (w143:cluster{"x0":dbl, "dx":dbl, "y":sgl[]}[])
        n50 = To Variant(anything=w143) -> (Variant=w154:variant)
        n51 = call "EnQueue_Message_Single.vi"("Message Data"=w154, "Message"="CCDF_Disp", "Message_Queue"=w152) -> ()  [unwired: 7 in, 2 out]
      }
      frame "IQ_Disp" {
        n52 = call <vilib>:"RFmxSpecAn IQ Fetch Data.vi"("Instrument Handle In"=w162, "error in (no error)"=w161) -> ("Instrument Handle Out"=w160:refnum<k21>, "Data"=w155:cluster{"t0":dbl, "dt":dbl, "Y":csg[]}, "error out"=w159:errorcluster)  [unwired: 11 in]
        n53 = To Variant(anything=w155) -> (Variant=w158:variant)
        n54 = call "EnQueue_Message_Single.vi"("Message Data"=w158, "Message"="IQ_Disp", "Message_Queue"=w156) -> ()  [unwired: 7 in, 2 out]
      }
      frame "IMD_Data" {
        n55 = call-poly <vilib>:"RFmxSpecAn Spectrum Fetch.vi"("Instrument Handle In"=w168, "Selector String"=w163, "error in (no error)"=w167) -> ("Frequency Resolution (Hz)"=w172:dbl, "Instrument Handle Out"=w166:refnum<k21>, "Peak Amplitude"=w171:dbl, "Peak Frequency (Hz)"=w170:dbl, "error out"=w165:errorcluster)  [unwired: 8 in]
        n56 = Build Array(w172, w171, w170) -> (w169:dbl[])
        n57 = To Variant(anything=w169) -> (Variant=w174:variant)
        n58 = call "EnQueue_Message_Single.vi"("Message Data"=w174, "Message"="IMD_Data", "Message_Queue"=w164) -> ()  [unwired: 7 in, 2 out]
      }
      frame "IMD_Disp" {
        n59 = call-poly <vilib>:"RFmxSpecAn Spectrum Fetch.vi"("Instrument Handle In"=w180, "Selector String"=w175, "error in (no error)"=w179) -> ("Instrument Handle Out"=w177:refnum<k21>, "Spectrum"=w181:cluster{"x0":dbl, "dx":dbl, "y":sgl[]}, "error out"=w176:errorcluster)  [unwired: 10 in]
        n60 = To Variant(anything=w181) -> (Variant=w183:variant)
        n61 = call "EnQueue_Message_Single.vi"("Message Data"=w183, "Message"="IMD_Disp", "Message_Queue"=w178) -> ()  [unwired: 7 in, 2 out]
      }
      frame "SFDR_Data" {
        n62 = call-poly <vilib>:"RFmxSpecAn Spectrum Fetch.vi"("Instrument Handle In"=w188, "error in (no error)"=w187) -> ("Frequency Resolution (Hz)"=w192:dbl, "Instrument Handle Out"=w186:refnum<k21>, "Peak Amplitude"=w191:dbl, "Peak Frequency (Hz)"=w190:dbl, "error out"=w185:errorcluster)  [unwired: 9 in]
        n63 = Build Array(w192, w191, w190) -> (w189:dbl[])
        n64 = To Variant(anything=w189) -> (Variant=w194:variant)
        n65 = call "EnQueue_Message_Single.vi"("Message Data"=w194, "Message"="SFDR_Data", "Message_Queue"=w184) -> ()  [unwired: 7 in, 2 out]
      }
      frame "SFDR_Disp" {
        n66 = call-poly <vilib>:"RFmxSpecAn Spectrum Fetch.vi"("Instrument Handle In"=w199, "error in (no error)"=w198) -> ("Instrument Handle Out"=w196:refnum<k21>, "Spectrum"=w200:cluster{"x0":dbl, "dx":dbl, "y":sgl[]}, "error out"=w195:errorcluster)  [unwired: 11 in]
        n67 = To Variant(anything=w200) -> (Variant=w202:variant)
        n68 = call "EnQueue_Message_Single.vi"("Message Data"=w202, "Message"="SFDR_Disp", "Message_Queue"=w197) -> ()  [unwired: 7 in, 2 out]
      }
      frame "Harmonics_Data" {
        n69 = for {
          N: 3 -> [_]
          shift-right: [w217] -> w205
          shift-left: w207 -> [w224]
          shift-right: [w216] -> w204
          shift-left: w206 -> [w223]
          tunnel: w208 -> [w222]
          tunnel: [w215] -> w203 mode=indexing
          i -> [w214]
          n70 = Increment(x=w214) -> (x+1=w213:i32)
          n71 = Number To Decimal String(number=w213) -> (decimal integer string=w219:string)  [unwired: 1 in]
          n72 = Concatenate Strings(w222, "Harms" ("name (unnamed)"), w219) -> (w221:string)
          n73 = call <vilib>:"RFmxSpecAn Build Signal String.vi"("Signal Name"=w221, "Result Name"=w221) -> ("Selector String"=w218:string)  [unwired: 13 in]
          n74 = call-poly <vilib>:"RFmxSpecAn Spectrum Fetch.vi"("Instrument Handle In"=w224, "Selector String"=w218, "error in (no error)"=w223) -> ("Instrument Handle Out"=w217:refnum<k21>, "Peak Amplitude"=w215:dbl, "error out"=w216:errorcluster)  [unwired: 8 in, 2 out]
        }
        n75 = To Variant(anything=w203) -> (Variant=w212:variant)
        n76 = call "EnQueue_Message_Single.vi"("Message Data"=w212, "Message"="Harmonics_Data", "Message_Queue"=w210) -> ()  [unwired: 7 in, 2 out]
      }
      frame "Harmonics_Disp" {
        n77 = for {
          N: 3 -> [_]
          shift-right: [w239] -> w228
          shift-left: w230 -> [w242]
          shift-right: [w240] -> w227
          shift-left: w229 -> [w241]
          tunnel: w226 -> [w246]
          tunnel: [w237] -> w225 mode=indexing
          i -> [w236]
          n78 = Increment(x=w236) -> (x+1=w235:i32)
          n79 = Number To Decimal String(number=w235) -> (decimal integer string=w243:string)  [unwired: 1 in]
          n80 = Concatenate Strings(w246, "Harms" ("name (unnamed)"), w243) -> (w245:string)
          n81 = call <vilib>:"RFmxSpecAn Build Signal String.vi"("Signal Name"=w245, "Result Name"=w245) -> ("Selector String"=w238:string)  [unwired: 13 in]
          n82 = call-poly <vilib>:"RFmxSpecAn Spectrum Fetch.vi"("Instrument Handle In"=w242, "Selector String"=w238, "error in (no error)"=w241) -> ("Instrument Handle Out"=w239:refnum<k21>, "Spectrum"=w237:cluster{"x0":dbl, "dx":dbl, "y":sgl[]}, "error out"=w240:errorcluster)  [unwired: 10 in]
        }
        n83 = To Variant(anything=w225) -> (Variant=w234:variant)
        n84 = call "EnQueue_Message_Single.vi"("Message Data"=w234, "Message"="Harmonics_Disp", "Message_Queue"=w232) -> ()  [unwired: 7 in, 2 out]
      }
    }
  }
  "Instrument Handle out" <- w3
  "error out" <- w4
